vi "Enable PPSU.vi"() -> (0 "error Out":errorcluster, 1 "PPSU IP String":string, 2 "Device information array":string[][](array[string]), 3 "Device information":string[](array[string]))   [LabVIEW 2022 SP3]
uses:
  Controls/ALL Health.ctl
  6D_Global.vi
panel:
  out "Data of the initialized master":string[](array[string])
  out ".not. x?":bool
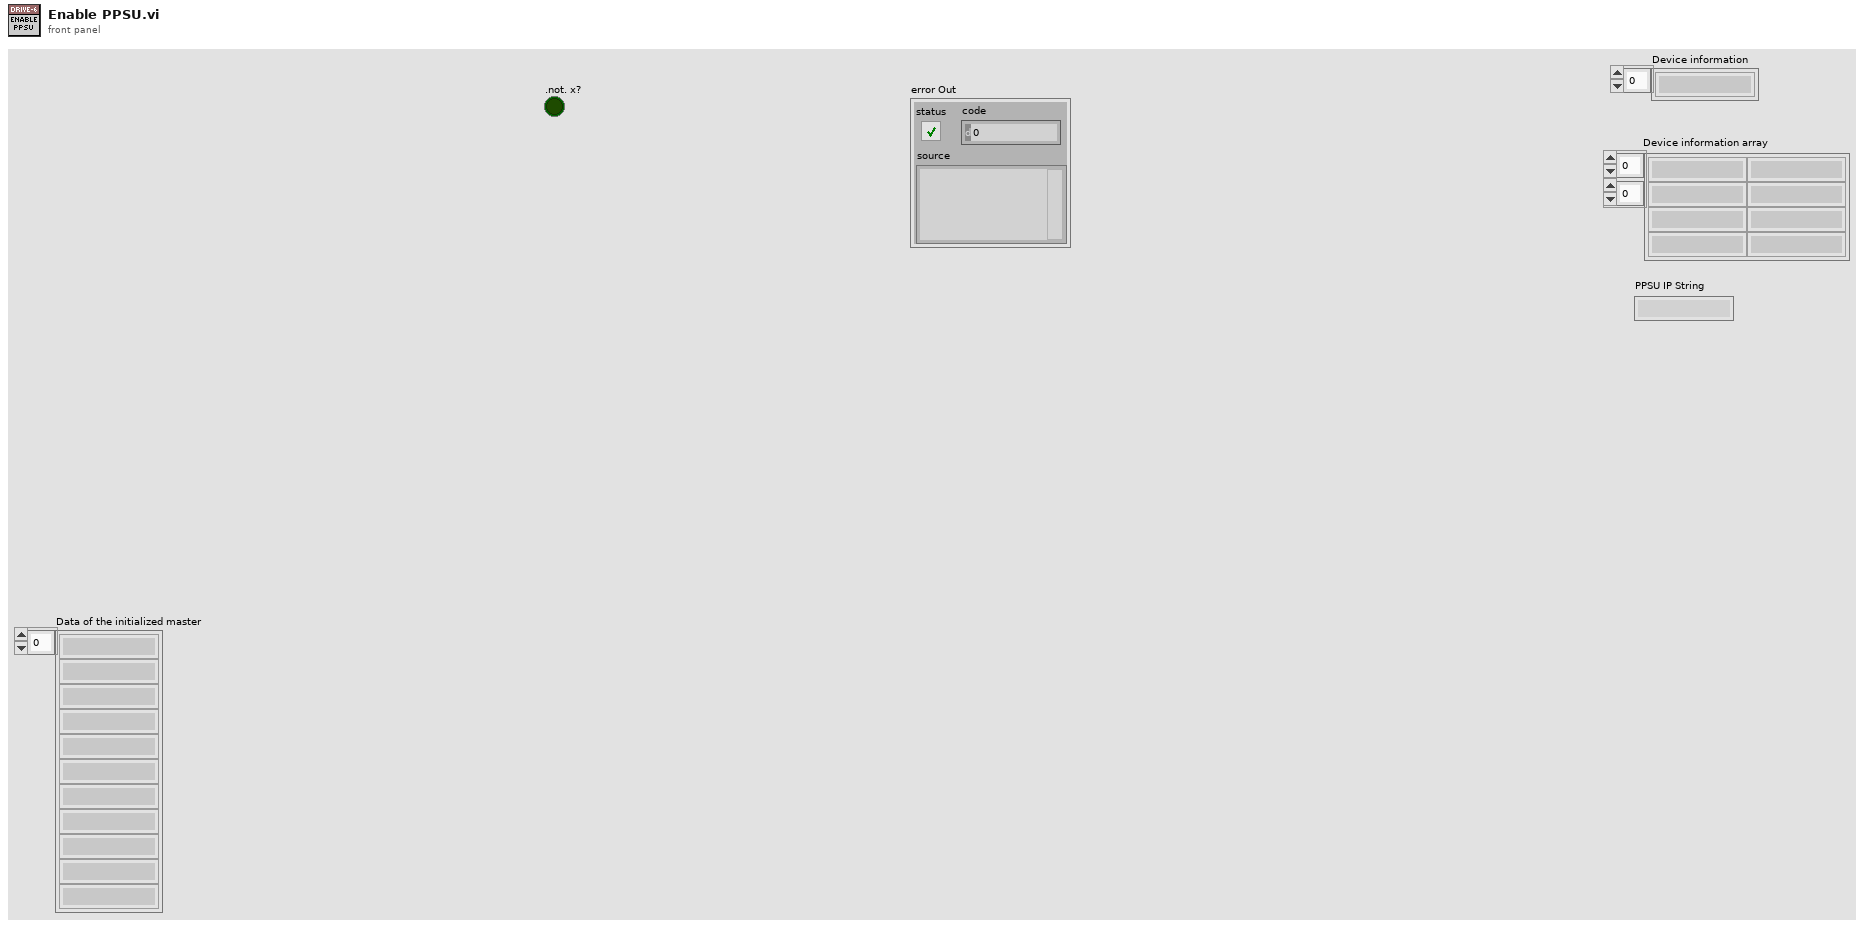
[diagram p1: front panel]
types:
  T1 = cluster{"Start ip":u8[], "Stop ip":u8[], "Port":u16}
  T2 = cluster{"Start IP":u8[], "Stop IP":u8[], "port":u16}
  T3 = typedef "ALL Health.ctl" = enum16{"AI HS", "AI Vibration HS", "AI Propulsion HS", "DO HS", "Datalog HS", "PPSU HS", "ETH_1 DAQ", "ETH_1 RTD", "ETH_2 DAQ", "ETH_2 RTD", "ETH_5 RTD"}
  T4 = enum16{"Init", "Read 'All'", "Read 'n'", "Read '1'", "Write '1'", "Write 'n'", "Write 'All'"}
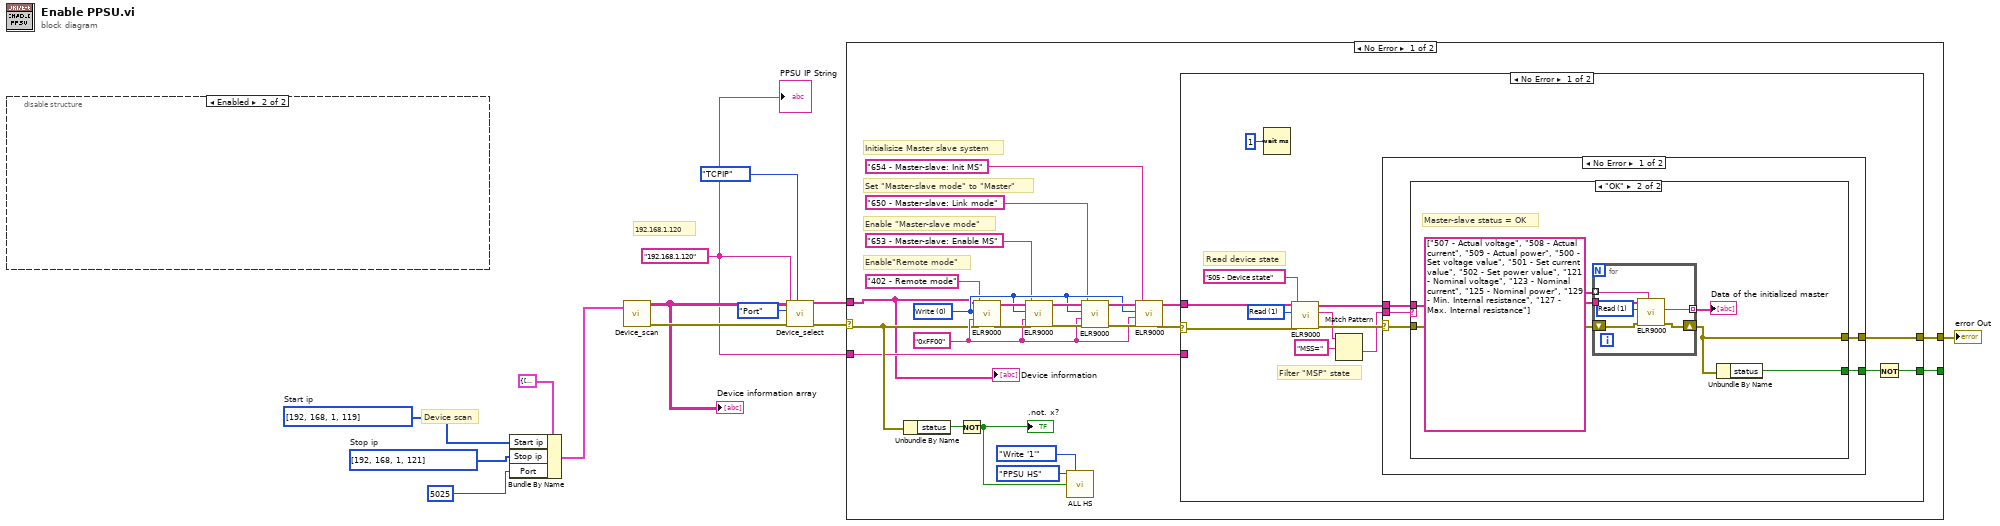
[diagram p0: block diagram]
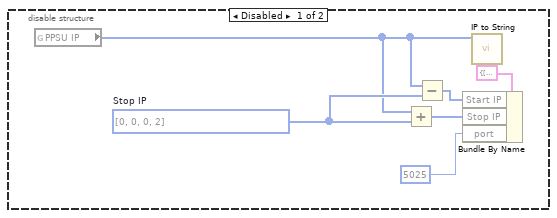
[diagram p2: hidden frame]
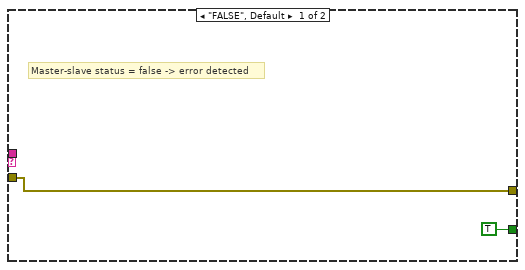
[diagram p3: hidden frame]
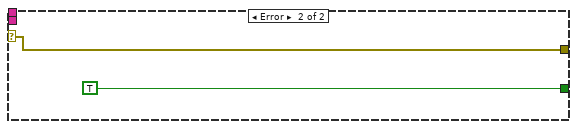
[diagram p4: hidden frame]
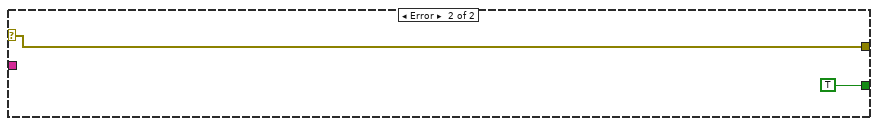
[diagram p5: hidden frame]
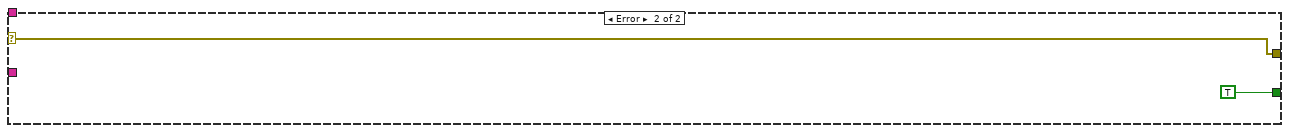
[diagram p6: hidden frame]
diagram:
  w2 = "192.168.1.120" ("PPSU IP String")
  w4 = u8[] [192, 168, 1, 121]  # Stop ip
  w5 = u8[] [192, 168, 1, 119]  # Start ip
  # "192.168.1.120"
  # "Device scan"
  n1 = disable-structure shown="Enabled" {
    frame Disabled {
      w15 = u8[] [0, 0, 0, 2]  # Stop IP
      n2 = global read "6D_Global.vi" "PPSU IP"() -> (w14:u8[])
      n3 = Add(x=w14, y=w15) -> (x+y=w17:u8[])
      n4 = Subtract(x=w14, y=w15) -> (x-y=w16:u8[])
      n5 = Bundle By Name(cluster=T2 {"Start IP"=[], "Stop IP"=[], "port"=0}, "Start IP"=w16, "Stop IP"=w17, "port"=u16 5025) -> ()  [unwired: 1 out]
      n6 = call "IP to String.vi"("Start IP"=w14) -> ()  [unwired: 10 in, 1 out]
    }
    frame Enabled {
    }
  }
  n7 = Bundle By Name(cluster=T1 {"Start ip"=[], "Stop ip"=[], "Port"=1001} ("IP adress(es) Cluster"), "Start ip"=w5, "Stop ip"=w4, "Port"=u16 5025) -> (w3:T1)
  n8 = call <vilib>:"Device_scan.vi"("IP settings"=w3) -> ("Device information array"=w8:string[][], "error out"=w9:errorcluster)  [unwired: 1 in, 2 out]
  "Device information array" <- w8
  n9 = call <vilib>:"Device_select.vi"("Reference"=enum16{"ASRL/COM", "GPIB", "TCPIP"}."TCPIP", "error in (no error)"=w9, "Alias"=w2, "Open by"=enum16{"Device Node", "Serial number", "Port"}."Port", "Device information array"=w8) -> ("error out"=w12:errorcluster, "Device information"=w13:string[])  [unwired: 2 in]
  n10 = case shown="No Error" w12 {
    selector: w12 -> [w27 w79]
    tunnel: [w38 TRUE] -> _
    tunnel: w13 -> [w20 _]
    tunnel: w2 -> [w25 _]
    tunnel: [w24 w79] -> w10
    frame No Error {
      w32 = u8 0 items=["Write", "Read"] ("Access")
      w33 = "0xFF00" ("Value")
      # "Initialisize Master slave system"
      # "Set \"Master-slave mode\" to \"Master\""
      # "Enable \"Master-slave mode\""
      # "Enable\"Remote mode\""
      n11 = Unbundle By Name(w27) -> ("status"=w26:bool)
      n12 = Not(x=w26) -> (.not. x?=w21:bool)
      ".not. x?" <- w21
      n13 = call <vilib>:"ELR9000.vi"("Command list"="402 - Remote mode", "Error in"=w27, "Value"=w33, "Access"=w32, "Device information in"=w20) -> ("Error out"=w40:errorcluster, "Device information out"=w39:string[])  [unwired: 1 in, 2 out]
      n14 = call <vilib>:"ELR9000.vi"("Command list"="653 - Master-slave: Enable MS", "Error in"=w40, "Value"=w33, "Access"=w32, "Device information in"=w39) -> ("Error out"=w37:errorcluster, "Device information out"=w34:string[])  [unwired: 1 in, 2 out]
      n15 = call "ALL HS.vi"("Loop"=ALL_Health."PPSU HS", "Option"=T4."Write '1'", "Status"=w21) -> ()  [unwired: 10 in, 3 out]
      n16 = call <vilib>:"ELR9000.vi"("Command list"="650 - Master-slave: Link mode", "Error in"=w37, "Value"=w33, "Access"=w32, "Device information in"=w34) -> ("Error out"=w36:errorcluster, "Device information out"=w35:string[])  [unwired: 1 in, 2 out]
      n17 = call <vilib>:"ELR9000.vi"("Command list"="654 - Master-slave: Init MS", "Error in"=w36, "Value"=w33, "Access"=w32, "Device information in"=w35) -> ("Error out"=w42:errorcluster, "Device information out"=w41:string[])  [unwired: 1 in, 2 out]
      n18 = case shown="No Error" w42 {
        selector: w42 -> [w45 w77]
        tunnel: w41 -> [w44 _]
        tunnel: [w55 TRUE] -> w38
        tunnel: w25 -> [_ _]
        tunnel: [w43 w77] -> w24
        frame No Error {
          w54 = u8 1 items=["Write", "Read"] ("Access")
          # "Read device state"
          # "Filter \"MSP\" state"
          n19 = Wait (ms)(milliseconds to wait=u32 1 ("Zu wartende ms")) -> ()  [unwired: 1 out]
          n20 = call <vilib>:"ELR9000.vi"("Command list"="505 - Device state", "Error in"=w45, "Access"=w54, "Device information in"=w44) -> ("Error out"=w53:errorcluster, "Read data"=w51:string, "Device information out"=w52:string[])  [unwired: 2 in, 1 out]
          n21 = Match Pattern(string=w51, regular expression="MSS=" ("regulärer Ausdruck")) -> (after substring=w48:string)  [unwired: 1 in, 3 out]
          n22 = case shown="No Error" w53 {
            selector: w53 -> [w58 w75]
            tunnel: w48 -> [w60 _]
            tunnel: w52 -> [w59 _]
            tunnel: [w57 TRUE] -> w49
            tunnel: [w56 w75] -> w43
            frame No Error {
              n23 = case shown="\"OK\"" w60 {
                tunnel: w59 -> [_ w67]
                tunnel: w58 -> [w61 w66]
                tunnel: [TRUE w65] -> w57
                tunnel: [w61 w63] -> w56
                frame "FALSE", Default {
                  # "Master-slave status = false -> error detected"
                }
                frame "OK" {
                  # "Master-slave status = OK"
                  n24 = for {
                    tunnel: w67 -> [w74]
                    tunnel: string[] ["507 - Actual voltage", "508 - Actual current", "509 - Actual power", "500 - Set voltage value", "501 - Set current value", "502 - Set power value", "121 - Nominal voltage", "123 - Nominal current", "125 - Nominal power", "129 - Min. Internal resistance", "127 - Max. Internal resistance"] -> [w72] mode=indexing
                    shift-right: [w70] -> w63
                    shift-left: w66 -> [w71]
                    tunnel: [w69] -> w68 mode=indexing
                    w73 = u8 1 items=["Write", "Read"] ("Access")
                    n25 = call <vilib>:"ELR9000.vi"("Command list"=w72, "Error in"=w71, "Access"=w73, "Device information in"=w74) -> ("Error out"=w70:errorcluster, "Read data"=w69:string)  [unwired: 2 in, 2 out]
                  }
                  "Data of the initialized master" <- w68
                  n26 = Unbundle By Name(w63) -> ("status"=w65:bool)
                }
              }
            }
            frame Error {
            }
          }
          n27 = Not(x=w49) -> (.not. x?=w55:bool)
        }
        frame Error {
        }
      }
      "Device information" <- w20
    }
    frame Error {
    }
  }
  "error Out" <- w10
  "PPSU IP String" <- w2
